vi "custom stimulus.vi"() -> ()   [LabVIEW 2014]
uses:
  <vilib>/userdefined/High Color/IMAQdx.ctl
  <vilib>/Utility/file.llb/Read From Spreadsheet File (DBL).vi
  <vilib>/Utility/file.llb/Write To Spreadsheet File (DBL).vi
  <vilib>/Utility/file.llb/Write To Spreadsheet File (string).vi
  <vilib>/vision/driver/NI_Vision_Acquisition_Software.lvlib
panel:
  in  "Wait between stimuli (frames)":i32
  in  "Trials Per Voltage":i32
  in  "Start Recording":bool
  in  "Min Voltage":dbl
  in  "Frames":i32
  out "Error":string
  out "Save Directory":path
  out "Buffer Number Out":u32
  out "Image":T1(plugin-control)
  in  "stop":bool
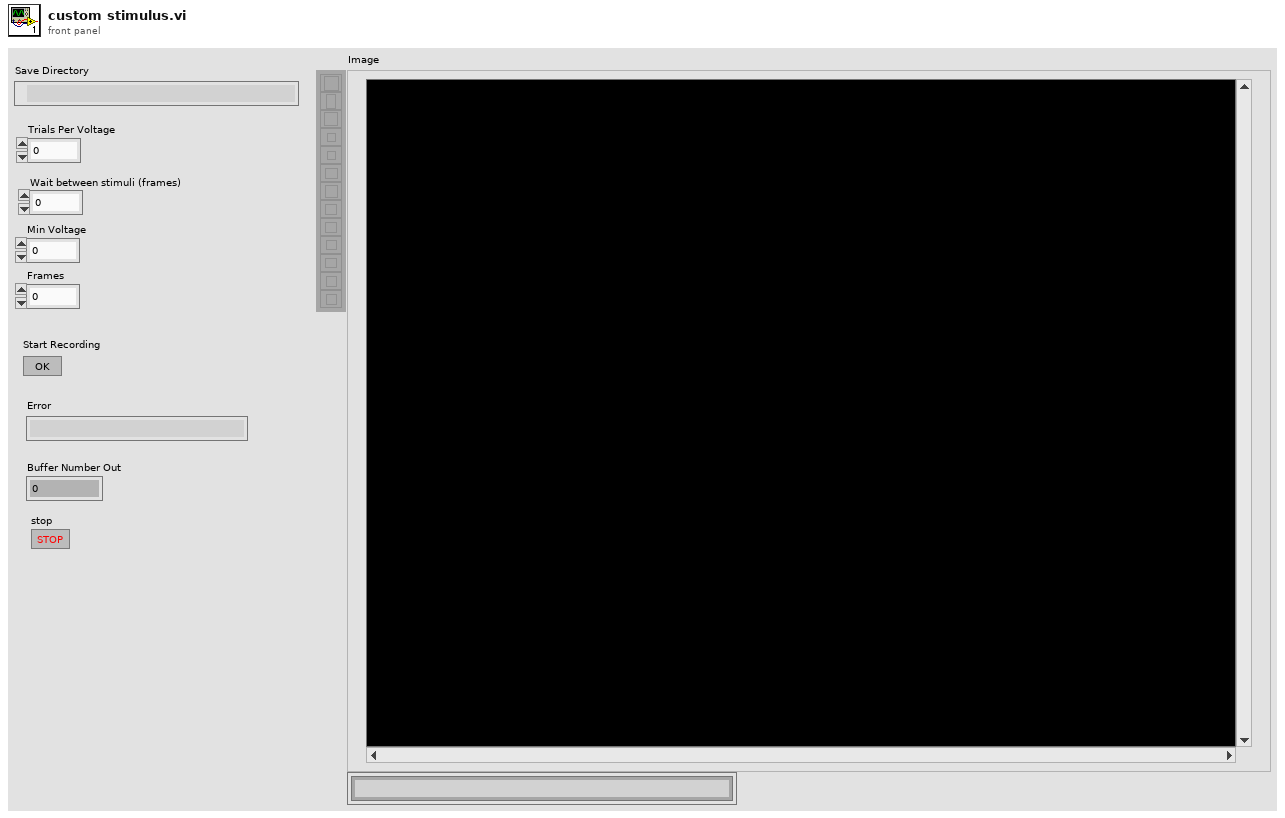
[diagram p1: front panel]
types:
  T1 = typedef "IMAQ Image.ctl" = refnum<image>
  T2 = typedef "IMAQdx.ctl" = refnum<k21>
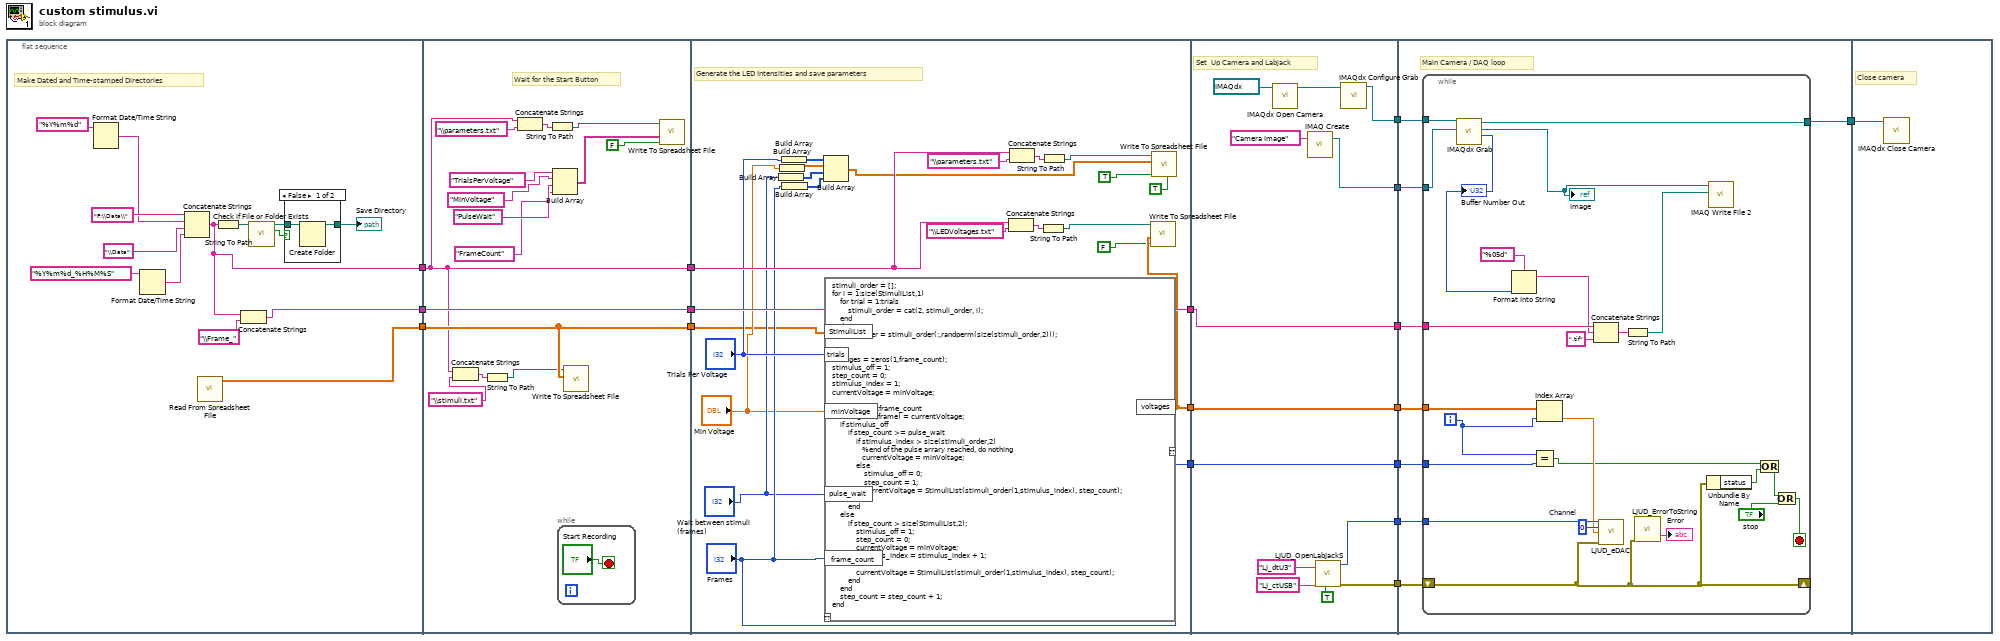
[diagram p0: block diagram]
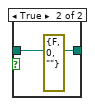
[diagram p2: hidden frame]
diagram:
  n1 = flat-sequence {
    tunnel: [w21] -> w6
    tunnel: [w19] -> w4
    tunnel: [w18] -> w1
    tunnel: w6 -> [w49]
    tunnel: [w49] -> w5
    tunnel: w4 -> [w39]
    tunnel: [w39] -> w3
    tunnel: [w41] -> w2
    tunnel: w1 -> [w41]
    tunnel: w5 -> [w70]
    tunnel: [w70] -> w11
    tunnel: [w68] -> w9
    tunnel: ["Frames"] -> w8
    tunnel: w3 -> [w62]
    tunnel: w2 -> [w53]
    tunnel: w11 -> [w80]
    tunnel: [w82] -> w17
    tunnel: [w81] -> w16
    tunnel: [w80] -> w15
    tunnel: [w76] -> w13
    tunnel: [w75] -> w12
    tunnel: [w74] -> w10
    tunnel: w9 -> [w74]
    tunnel: w8 -> [w73]
    tunnel: [w73] -> w7
    tunnel: w17 -> [w93]
    tunnel: w16 -> [w92]
    tunnel: w15 -> [w91]
    tunnel: [w90] -> w14
    tunnel: w13 -> [w89]
    tunnel: w12 -> [w88]
    tunnel: w10 -> [w87]
    tunnel: w7 -> [w86]
    tunnel: w14 -> [w118]
    frame #0 {
      # "Make Dated and Time-stamped Directories"
      n2 = Format Date/Time String(time format string (%c)="%Y%m%d") -> (date/time string=w22:string)  [unwired: 2 in]
      n3 = Format Date/Time String(time format string (%c)="%Y%m%d_%H%M%S") -> (date/time string=w26:string)  [unwired: 2 in]
      n4 = Concatenate Strings("F:\\Data\\", w22, "\\Data", w26) -> (w19:string)
      n5 = call-poly <vilib>:"Read From Spreadsheet File.vi"() -> ("all rows"=w18:dbl[][])  [unwired: 7 in, 4 out]
      n6 = String To Path(string=w19) -> (path=w25:path)
      n7 = Concatenate Strings(w19, "\\Frame_") -> (w21:string)
      n8 = call <vilib>:"Check if File or Folder Exists.vi"("path"=w25) -> ("file or folder exists?"=w30:bool, "dup path"=w29:path)  [unwired: 8 in, 1 out]
      n9 = case shown="False" w30 {
        tunnel: [w32 w34] -> w24
        tunnel: w29 -> [w33 w34]
        frame False {
          n10 = Create Folder(path (use dialog)=w33) -> (created path=w32:path)  [unwired: 2 in, 2 out]
        }
        frame True {
          (unwired) errorcluster {"status"=FALSE, "code"=0, "source"=""} ("error out")
        }
      }
      "Save Directory" <- w24
    }
    frame #1 {
      # "Wait for the Start Button"
      n11 = Concatenate Strings(w39, "\\stimuli.txt") -> (w40:string)
      n12 = String To Path(string=w40) -> (path=w37:path)
      n13 = Concatenate Strings(w39, "\\parameters.txt") -> (w48:string)
      n14 = String To Path(string=w48) -> (path=w47:path)
      n15 = Build Array("TrialsPerVoltage", "MinVoltage", "PulseWait", "FrameCount") -> (w44:string[])
      n16 = while {
        stop <- "Start Recording" stop-if-true
      }
      n17 = call-poly <vilib>:"Write To Spreadsheet File.vi"("2D data"=w41, "file path (dialog if empty)"=w37) -> ()  [unwired: 6 in, 1 out]
      n18 = call-poly <vilib>:"Write To Spreadsheet File.vi"("append to file? (new file:F)"=FALSE, "1D data"=w44, "file path (dialog if empty)"=w47) -> ()  [unwired: 5 in, 1 out]
    }
    frame #2 {
      # "Generate the LED Intensities and save parameters"
      n19 = Build Array("Wait between stimuli (frames)") -> (w52:i32[])
      n20 = Build Array("Min Voltage") -> (w54:dbl[])
      n21 = Build Array("Trials Per Voltage") -> (w60:i32[])
      n22 = Build Array("Frames") -> (w51:i32[])
      n23 = Build Array(w60, w54, w52, w51) -> (w58:dbl[][])
      n24 = script code="stimuli_order = [];\nfor i = 1:size(StimuliList,1)\n    for trial = 1:trials\n        stimuli_order = cat(2, stimuli_order, i);\n    end\nend\nstimuli_order = stimuli_order(:,randperm(size(stimuli_order,2)));\n\n\nvoltages = zeros(1,frame_count);\nstimulus_off = 1;\nstep_count = 0;\nstimulus_index = 1;\ncurrentVoltage = minVoltage;\n\nfor frame = 1:frame_count\n    voltages(1,frame) = currentVoltage;\n    if stimulus_off\n        if step_count >= pulse_wait\n            if stimulus_index > size(stimuli_order,2)\n               %end of the pulse arrary reached, do nothing\n               currentVoltage = minVoltage;\n            else\n                stimulus_off = 0;\n                step_count = 1;\n                currentVoltage = StimuliList(stimuli_order(1,stimulus_index), step_count);\n            end\n        end\n    else\n        if step_count > size(StimuliList,2);\n            stimulus_off = 1;\n            step_count = 0;\n            currentVoltage = minVoltage;\n            stimulus_index = stimulus_index + 1;\n        else\n            currentVoltage = StimuliList(stimuli_order(1,stimulus_index), step_count);\n        end\n    end\n    step_count = step_count + 1;\nend"("frame_count"="Frames", "trials"="Trials Per Voltage", "minVoltage"="Min Voltage", "StimuliList"=w53, "pulse_wait"="Wait between stimuli (frames)") -> ("voltages"=w68:dbl[])  [unwired: 1 in, 1 out]
      n25 = Concatenate Strings(w62, "\\LEDVoltages.txt") -> (w72:string)
      n26 = Concatenate Strings(w62, "\\parameters.txt") -> (w66:string)
      n27 = String To Path(string=w72) -> (path=w71:path)
      n28 = String To Path(string=w66) -> (path=w65:path)
      n29 = call-poly <vilib>:"Write To Spreadsheet File.vi"("append to file? (new file:F)"=FALSE, "1D data"=w68, "file path (dialog if empty)"=w71) -> ()  [unwired: 5 in, 1 out]
      n30 = call-poly <vilib>:"Write To Spreadsheet File.vi"("transpose? (no:F)"=TRUE, "append to file? (new file:F)"=TRUE, "2D data"=w58, "file path (dialog if empty)"=w65) -> ()  [unwired: 4 in, 1 out]
    }
    frame #3 {
      # "Set  Up Camera and Labjack"
      n31 = call <vilib>:"IMAQdx Open Camera.vi"("Session In"=T2 "cam0") -> ("Session Out"=w84:T2)  [unwired: 9 in, 1 out]
      n32 = call "IMAQ Create"("Image Name"="Camera Image") -> ("New Image"=w81:T1)  [unwired: 4 in, 1 out]
      n33 = call "LJUD_OpenLabJackS.vi"("FirstFound"=TRUE, "ConnectionType"="LJ_ctUSB", "DeviceType"="LJ_dtU3") -> ("error out"=w75:errorcluster, "Handle"=w76:i32)  [unwired: 6 in, 1 out]
      n34 = call <vilib>:"IMAQdx Configure Grab.vi"("Session In"=w84) -> ("Session Out"=w82:T2)  [unwired: 9 in, 1 out]
    }
    frame #4 {
      # "Main Camera / DAQ loop"
      n35 = while {
        tunnel: w93 -> [w117]
        tunnel: [w116] -> w90
        tunnel: w92 -> [w115]
        tunnel: w91 -> [w113]
        tunnel: w89 -> [w106]
        shift-right: [w103] -> _
        shift-left: w88 -> [w103]
        tunnel: w87 -> [w95]
        tunnel: w86 -> [w94]
        i -> [w96]
        stop <- w105 stop-if-true
        w102 = 0  # Channel
        n36 = call <vilib>:"IMAQdx Grab.vi"("Image In"=w115, "Session In"=w117) -> ("Buffer Number Out"=w109:u32, "Image Out"=w114:T1, "Session Out"=w116:T2)  [unwired: 6 in, 1 out]
        "Image" <- w114
        "Buffer Number Out" <- w109
        n37 = Format Into String(format string="%05d" ("string"), w109) -> (resulting string=w108:string)  [unwired: 2 in, 1 out]
        n38 = Equal?(x=w96, y=w94) -> (x = y?=w98:bool)
        n39 = Index Array(array=w95, index=w96) -> (element=w100:dbl)
        n40 = Concatenate Strings(w113, w108, ".tif" ("string")) -> (w111:string)
        n41 = call "LJUD_eDAC.vi"("Handle In"=w106, "Channel"=w102, "Voltage"=w100, "error in"=w103) -> ()  [unwired: 10 in, 2 out]
        n42 = String To Path(string=w111) -> (path=w110:path)
        n43 = call "LJUD_ErrorToString.vi"("error in"=w103) -> ("String"=→"Error":string)  [unwired: 10 in]
        n44 = Unbundle By Name(w103) -> ("status"=w99:bool)
        n45 = call-poly "IMAQ Write File 2"("File Path"=w110, "Image"=w114) -> ()  [unwired: 8 in, 2 out]
        n46 = Or(x=w98, y=w99) -> (x .or. y?=w97:bool)
        n47 = Or(x=w97, y="stop") -> (x .or. y?=w105:bool)
      }
    }
    frame #5 {
      # "Close camera"
      n48 = call <vilib>:"IMAQdx Close Camera.vi"("Session In"=w118) -> ()  [unwired: 10 in, 1 out]
    }
  }
